vi "test_232_imu_MW-AHRSv1_3d.vi"() -> ()   [LabVIEW 2019]
uses:
  <vilib>/picture/3D Picture Control/NI_3D Picture Control.lvlib
  <vilib>/picture/3D Picture Control/Object/Create Object (name).vi
  <vilib>/Instr/_visa.llb/VISA Configure Serial Port (Instr).vi
  Ctrl/cmd_imu.ctl
panel:
  in  "탭 컨트롤":enum32{"3d ui"}(tab)
  out "3D Picture":refnum<vi>(3d-picture)
  out "dir":picture
  out "heading":dbl format="%.1f"
  in  "baud rate":u32=115200 caption="rate"
  in  "Port":refnum<visa-resource-name>="COM24"
  in  "w-data":string="ang"
  in  "offset":dbl
  in  "reset":bool
  out "error out":errorcluster caption="에러 출력"
  in  "w":bool
  out "r buff":u32(graph)
  in  "정지":bool
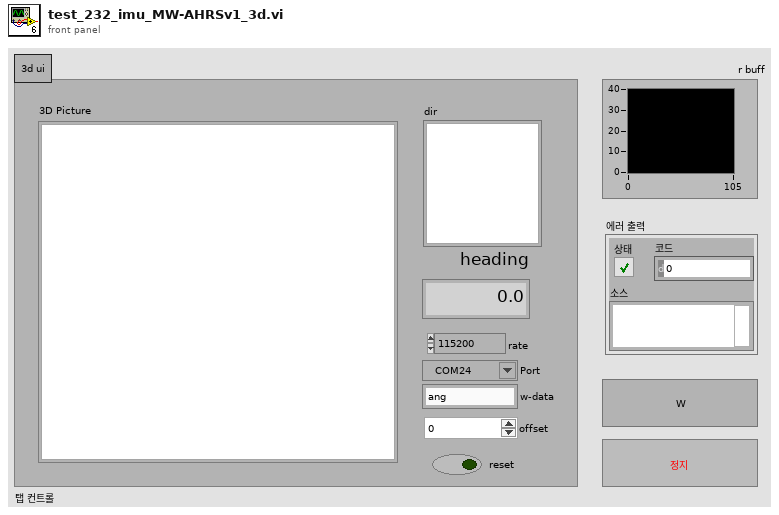
[diagram p1: front panel]
types:
  T1 = typedef "cmd_imu.ctl" = enum16{"ini", "write", "read"}
  T2 = cluster{"angle":dbl[], "acc":dbl[], "mag":dbl[], "gyr":dbl[]}
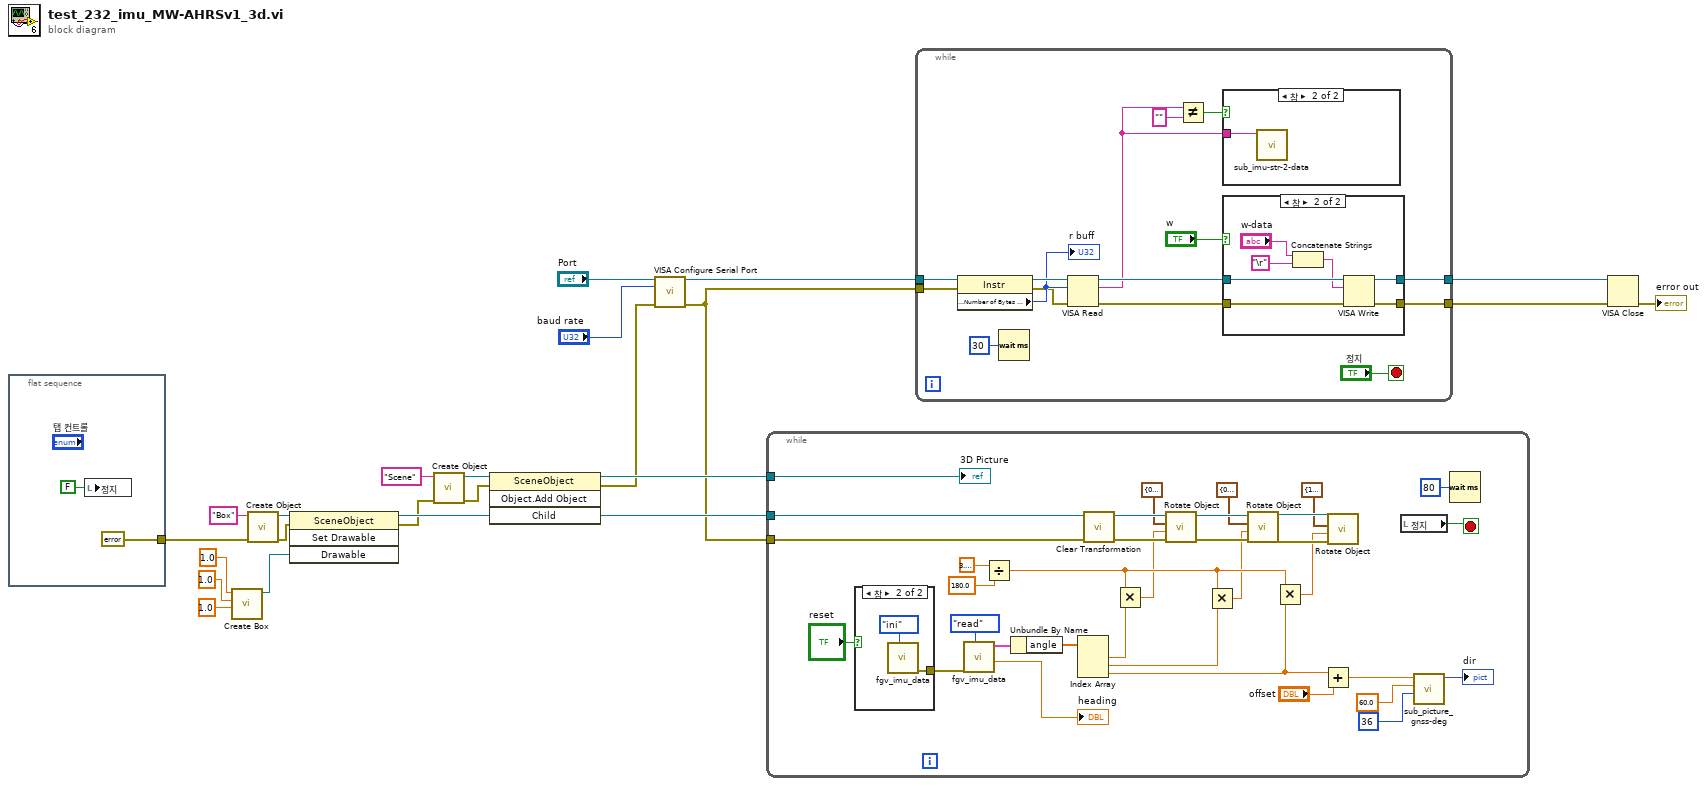
[diagram p0: block diagram]
diagram:
  n1 = flat-sequence {
    tunnel: [errorcluster {"status"=FALSE, "code"=0, "source"=""} ("error in (no error)")] -> w4
    frame #0 {
      n2 = local write "정지"(FALSE ("정지")) -> ()
    }
  }
  n3 = call <vilib>:"Create Box.vi"("Length Z"=sgl 1.0, "Length Y"=sgl 1.0, "Length X"=sgl 1.0) -> ("New Box Refnum"=w13:refnum<vi>)  [unwired: 7 in, 1 out]
  n4 = call-poly <vilib>:"Create Object.vi"("error in (no error)"=w4, "Name"="Box") -> ("error out"=w12:errorcluster, "Scene:New Object"=w11:refnum<vi>)  [unwired: 8 in]
  n5 = invoke class="SceneObject" method="Set Drawable"(reference=w11, error in=w12, "Drawable"=w13) -> (reference out=w17:refnum<vi>, error out=w3:errorcluster)  [unwired: 1 in, 2 out]
  n6 = call-poly <vilib>:"Create Object.vi"("error in (no error)"=w3, "Name"="Scene") -> ("error out"=w16:errorcluster, "Scene:New Object"=w15:refnum<vi>)  [unwired: 8 in]
  n7 = invoke class="SceneObject" method="Object.Add Object"(reference=w15, error in=w16, "Child"=w17) -> (reference out=w6:refnum<vi>, error out=w2:errorcluster, "Child"=w5:refnum<vi>)  [unwired: 1 in, 1 out]
  n8 = call-poly "VISA Configure Serial Port"("VISA resource name"="Port", "baud rate (9600)"="baud rate", "error in (no error)"=w2) -> ("VISA resource name out"=w21:refnum<visa-resource-name>, "error out"=w1:errorcluster)  [unwired: 11 in]
  n9 = while {
    tunnel: w6 -> [w45]
    tunnel: w5 -> [w59]
    tunnel: w1 -> [w36]
    stop <- w42 stop-if-true
    n10 = case shown="참" "reset" {
      tunnel: [_ w60] -> w27
      frame False {
      }
      frame True {
        n11 = call "fgv_imu_data.vi"("cmd"=cmd_imu."ini") -> ("error out"=w60:errorcluster)  [unwired: 7 in, 3 out]
      }
    }
    n12 = call "fgv_imu_data.vi"("cmd"=cmd_imu."read", "error in"=w27) -> ("heading"=→"heading":dbl, "IMD data out"=w40:T2)  [unwired: 6 in, 2 out]
    n13 = Divide(x=3.141592653589793, y=180.0) -> (x/y=w47:dbl)
    n14 = Unbundle By Name(w40) -> ("angle"=w39:dbl[])
    n15 = Index Array(array=w39) -> (element #1=w38:dbl, element #2=w37:dbl, element #3=w32:dbl)  [unwired: 3 in]
    n16 = call <vilib>:"Clear Transformation.vi"("error in (no error)"=w36, "Object Refnum In"=w59) -> ("error out"=w55:errorcluster, "Object Refnum Out"=w56:refnum<vi>)  [unwired: 8 in]
    n17 = Multiply(x=w47, y=w38) -> (x*y=w44:dbl)
    n18 = call <vilib>:"Rotate Object.vi"("error in (no error)"=w55, "Angle"=w44, "Axis"=cluster{"X":sgl, "Y":sgl, "Z":sgl} {"X"=0.0, "Y"=1.0, "Z"=0.0}, "Scene.Object In"=w56) -> ("error out"=w57:errorcluster, "Scene.Object Out"=w58:refnum<vi>)  [unwired: 6 in]
    n19 = Multiply(x=w47, y=w37) -> (x*y=w43:dbl)
    n20 = call <vilib>:"Rotate Object.vi"("error in (no error)"=w57, "Angle"=w43, "Axis"=cluster{"X":sgl, "Y":sgl, "Z":sgl} {"X"=0.0, "Y"=0.0, "Z"=1.0}, "Scene.Object In"=w58) -> ("error out"=w50:errorcluster, "Scene.Object Out"=w51:refnum<vi>)  [unwired: 6 in]
    n21 = Multiply(x=w47, y=w32) -> (x*y=w46:dbl)
    n22 = Add(x=w32, y="offset") -> (x+y=w31:dbl)
    n23 = call <vilib>:"Rotate Object.vi"("error in (no error)"=w50, "Angle"=w46, "Axis"=cluster{"X":sgl, "Y":sgl, "Z":sgl} {"X"=1.0, "Y"=0.0, "Z"=0.0}, "Scene.Object In"=w51) -> ()  [unwired: 6 in, 2 out]
    n24 = local read "정지"() -> (w42:bool)
    n25 = call "sub_picture_gnss-deg.vi"("radius"=i16 36, "Center"=60.0, "deg_gps"=w31) -> ("new picture"=→"dir":picture)  [unwired: 8 in]
    n26 = Wait (ms)(milliseconds to wait=u32 80 ("대기 시간 (ms)")) -> ()  [unwired: 1 out]
    "3D Picture" <- w45
  }
  n27 = while {
    tunnel: w1 -> [w71]
    tunnel: w21 -> [w70]
    tunnel: [w66] -> w19
    tunnel: [w65] -> w18
    stop <- "정지" stop-if-true
    n28 = property class="Instr"(reference=w70, error in=w71) -> (reference out=w75:refnum<visa-resource-name>, error out=w72:errorcluster, "Serial Settings:Number of Bytes at Serial Port"=w73:u32)
    "r buff" <- w73
    n29 = Wait (ms)(milliseconds to wait=u32 30 ("대기 시간 (ms)")) -> ()  [unwired: 1 out]
    n30 = VISA Read(VISA resource name=w75, byte count=w73, error in (no error)=w72) -> (VISA resource name out=w67:refnum<visa-resource-name>, read buffer=w62:string, error out=w68:errorcluster)  [unwired: 1 out]
    n31 = Not Equal?(x=w62, y="") -> (x != y?=w64:bool)
    n32 = case shown="참" w64 {
      tunnel: w62 -> [_ w77]
      frame False {
      }
      frame True {
        n33 = call "sub_imu-str-2-data.vi"("read buffer"=w77) -> ()  [unwired: 9 in, 2 out]
      }
    }
    n34 = case shown="참" "w" {
      tunnel: w67 -> [w79 w86]
      tunnel: [w79 w85] -> w66
      tunnel: w68 -> [w78 w84]
      tunnel: [w78 w83] -> w65
      frame False {
      }
      frame True {
        n35 = Concatenate Strings("w-data", "\r") -> (w80:string)
        n36 = VISA Write(VISA resource name=w86, write buffer=w80, error in (no error)=w84) -> (VISA resource name out=w85:refnum<visa-resource-name>, error out=w83:errorcluster)  [unwired: 1 out]
      }
    }
  }
  n37 = VISA Close(VISA resource name=w19, error in (no error)=w18) -> (error out=→"error out":errorcluster)
